vi "Old RoboTaxi VI.vi"() -> ()   [LabVIEW 2022 SP3]
doc: "This example performs writes and reads on a serial port, as directed by the user. You can press the Write and Read buttons, and change the Read Count, while the example is running.\n\nThe parameters set for the serial port must match the parameters of the connected instrument or device. In this example, the Read Count parameter specifies the number of bytes that the serial port reads. If there were more bytes at the port than the specified number, those bytes would not be read. If there were less bytes at the port than the specified number, you would receive a timeout error.\n\nThis example expands upon the flow control options for XON and XOFF, allowing the user to choose those control characters. Also, the user can enable or disable a termination character. Some devices require a termination character in order to identify the end of command strings. Some devices send a termination character to signify the end of data to be read. This example shows how you can end the Read operation once a termination character is detected in the buffer and/or append a termination character at the end of the Write data."
uses:
  Serial - Settings.ctl
  Serial - XON-XOFF Characters.ctl
  Serial - ASCII Characters.ctl
  ESP32-PSOC-State Machine.ctl
  <vilib>/Instr/_visa.llb/VISA Flush IO Buffer Mask.ctl
  <vilib>/Instr/_visa.llb/VISA Configure Serial Port (Instr).vi
panel:
  in  "Stop Driving":bool
  in  "Right":bool
  in  "Left":bool
  in  "Backward":bool
  in  "Forward":bool
  in  "Manual":bool
  in  "Autonomous":bool
  in  "Track 2":bool
  in  "Track 1":bool
  out "error":bool
  out "Connected":bool
  out "Serial Settings:Number of Bytes at Serial Port":u32
  out "Response 2":string
  in  "Toggle LED":bool
  in  "Enum":T1
  in  "Termination Character":u8=10 format="%.0x"
  in  "End Write on Termination Character?":bool=TRUE
  in  "Stop":bool
  out "Read Count":u32=1000
  out "Response":string
  in  "XON/XOFF Characters":T2={"XON"=enum."DC1", "XOFF"=enum."DC3"}
  in  "Serial Settings":T4={"baud rate"=115200, "data bits"=8, "parity"=enum."None", "stop bits"=10, "flow control"=0} {"flow control" items=["None"=0, "XON/XOFF"=1, "RTS/CTS"=2, "DTR/DSR"=4]; "stop bits" items=["1.0"=10, "1.5"=15, "2.0"=20]; "data bits" min=5 max=8 step=1; "baud rate" items=["75"=75, "110"=110, "134"=134, "150"=150, "300"=300, "600"=600, "1200"=1200, "1800"=1800, "2400"=2400, "4800"=4800, "7200"=7200, "9600"=9600, "14400"=14400, "19200"=19200, "28800"=28800, "38400"=38400, "56000"=56000, "57600"=57600, "115200"=115200, "128000"=128000, "230400"=230400]}
  in  "End Read on Termination Character?":bool=TRUE
  in  "VISA resource name":refnum<visa-resource-name>="COM5"
  # "ESP32 Control"
  # "Track Selection"
  # "Driving Mode"
  # "Manual Override"
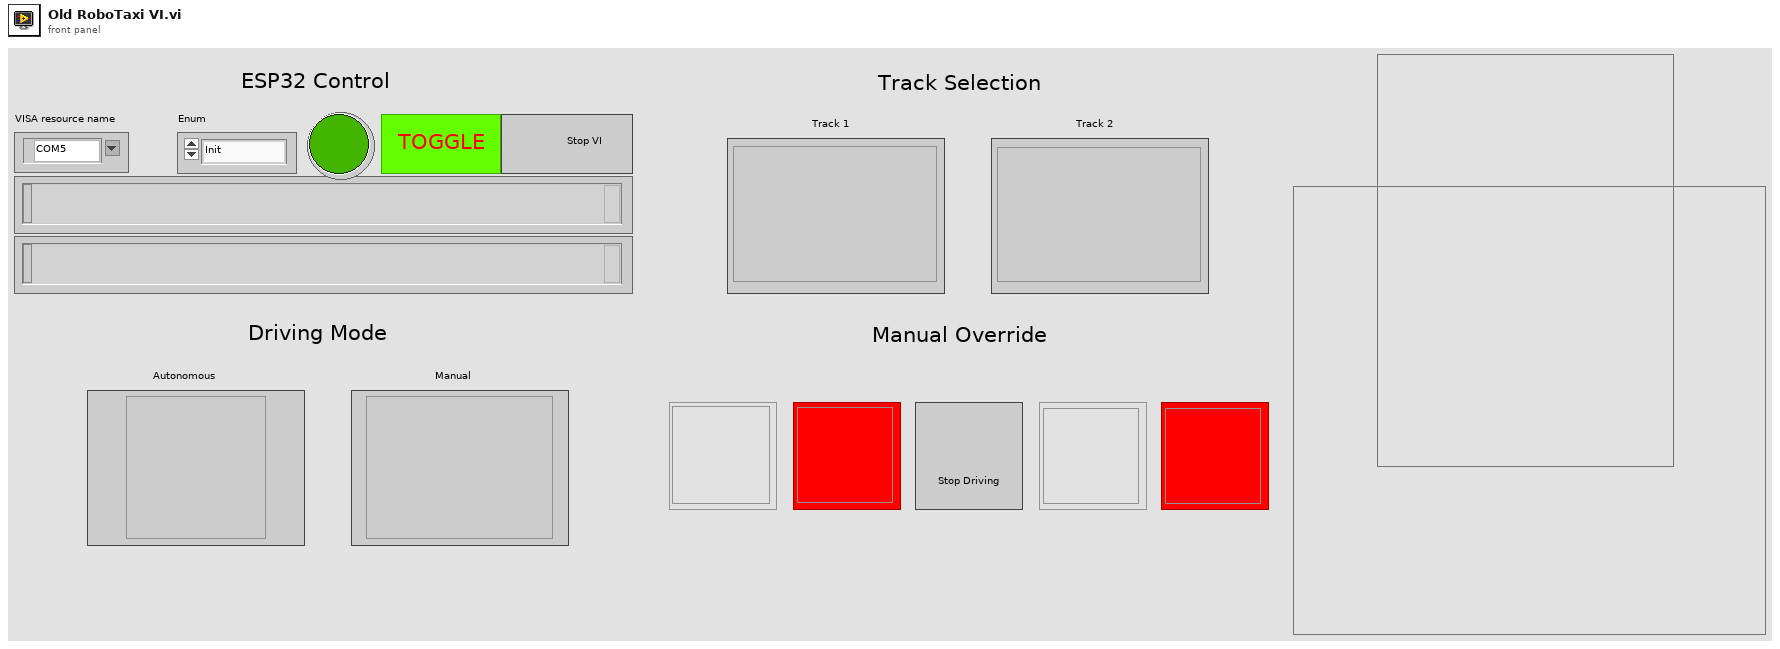
[diagram p1: front panel]
types:
  T1 = typedef "ESP32-PSOC-State Machine.ctl" = enum8{"Init", "Connect", "idle", "send", "wait", "receive", "que", "error", "exit"}
  T2 = typedef "Serial - XON-XOFF Characters.ctl" = cluster{"XON":T3, "XOFF":T3}
  T3 = typedef "Serial - ASCII Characters.ctl" = enum16{"NUL", "SOH", "STX", "ETX", "EOT", "ENQ", "ACK", "BEL", "BS", "HT", "LF", "VT", "FF", "CR", "SO", "SI", "DLE", "DC1", "DC2", "DC3", "DC4", "NAK", "SYN", "ETB", "CAN", "EM", "SUB", "ESC", "FS", "GS", "RS", "US", "SP", "!", "\"", "#", "$", "%", "&", "'", "(", ")", "*", "+", ",", "- (-)", ".", "/", "0", "1", "2", "3", "4", "5", "6", "7", "8", "9", ":", ";", "<", "=", ">", "?", "@", "A", "B", "C", "D", "E", "F", "G", "H", "I", "J", "K", "L", "M", "N", "O", "P", "Q", "R", "S", "T", "U", "V", "W", "X", "Y", "Z", "[", "\\", "]", "^", "_", "`", "a", "b", "c", "d", "e", "f", "g", "h", "i", "j", "k", "l", "m", "n", "o", "p", "q", "r", "s", "t", "u", "v", "w", "x", "y", "z", "{", "|", "}", "~"}
  T4 = typedef "Serial - Settings.ctl" = cluster{"baud rate":u32, "data bits":u16, "parity":enum16{"None", "Odd", "Even", "Mark", "Space"}, "stop bits":u16, "flow control":u16}
  T5 = typedef "VISA Flush IO Buffer Mask.ctl" = u16
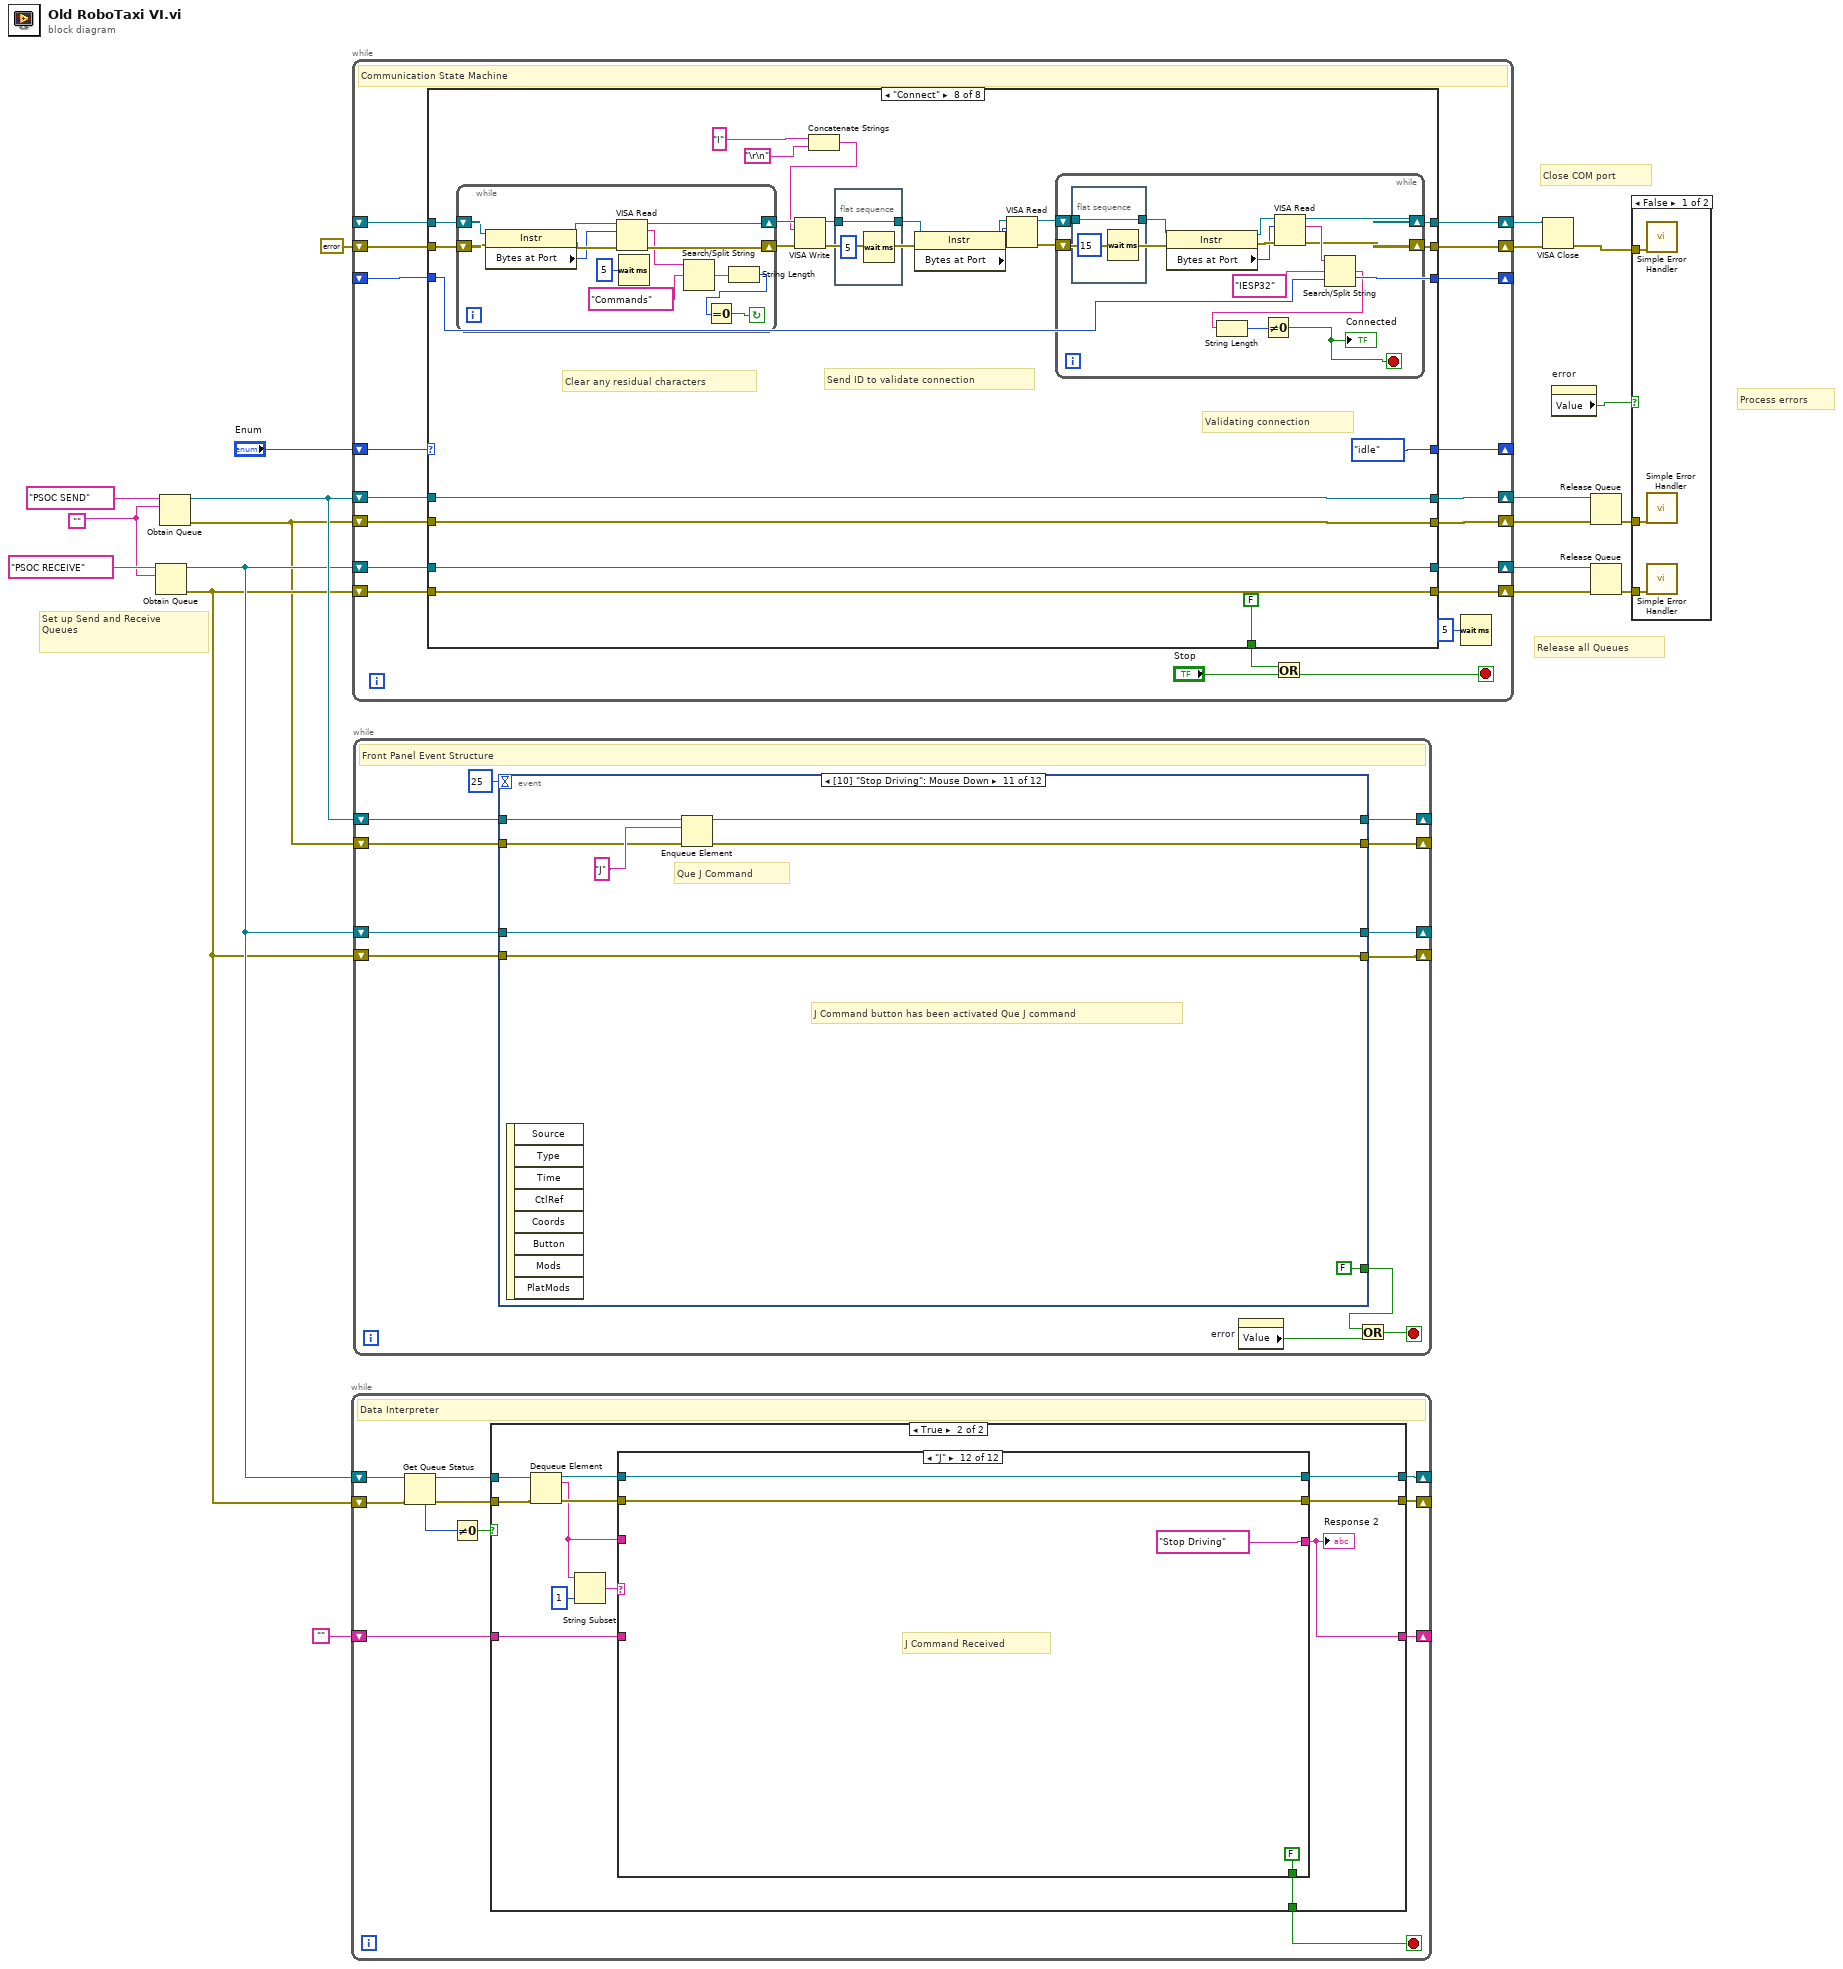
[diagram p0: block diagram]
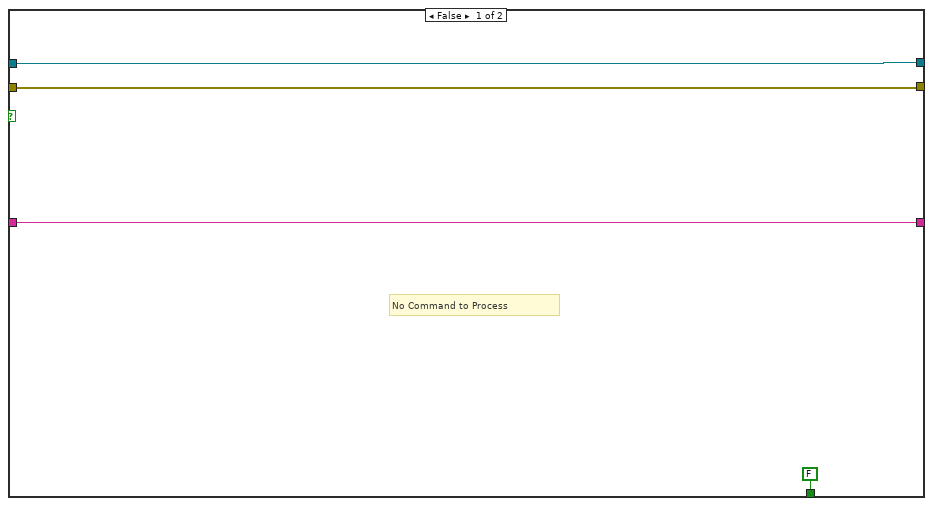
[diagram p3: hidden frame]
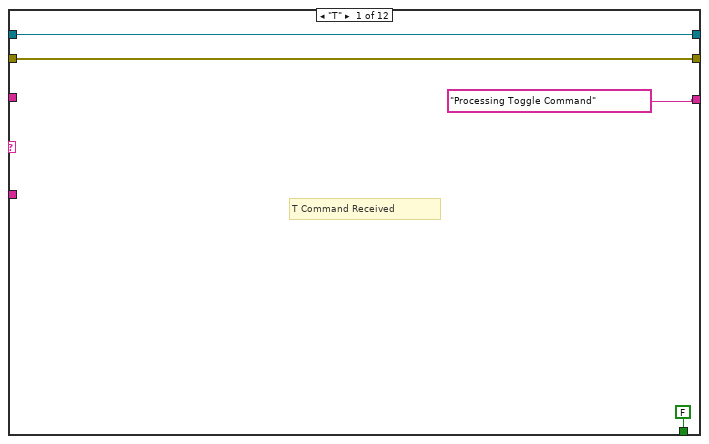
[diagram p4: hidden frame]
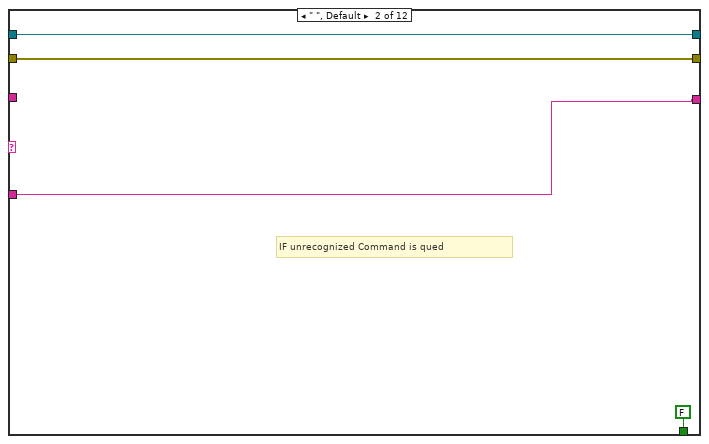
[diagram p5: hidden frame]
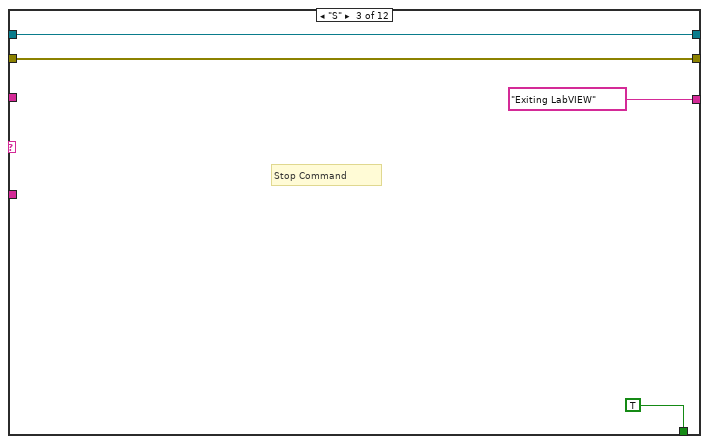
[diagram p6: hidden frame]
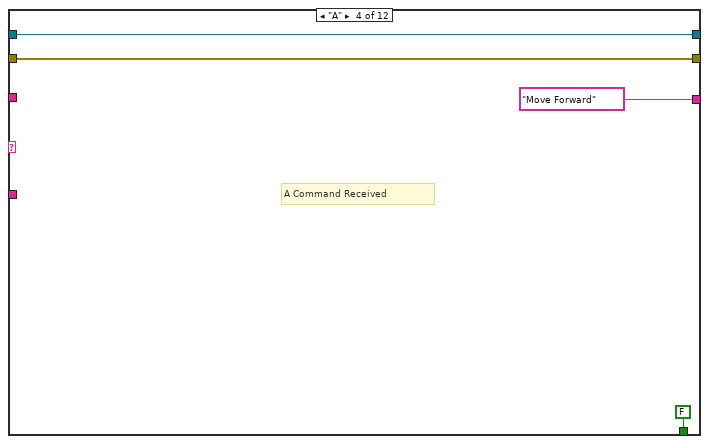
[diagram p7: hidden frame]
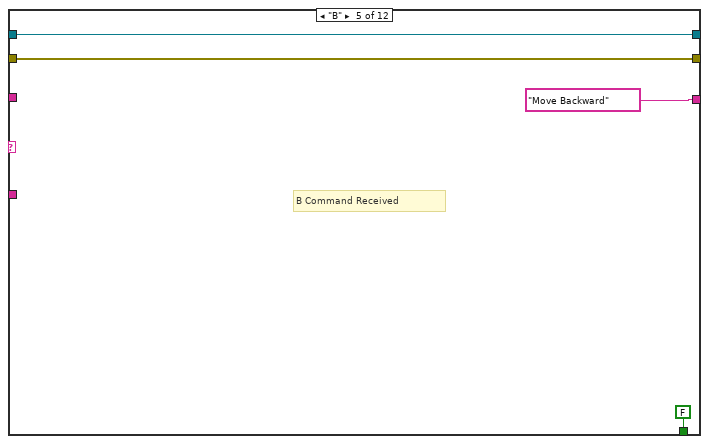
[diagram p8: hidden frame]
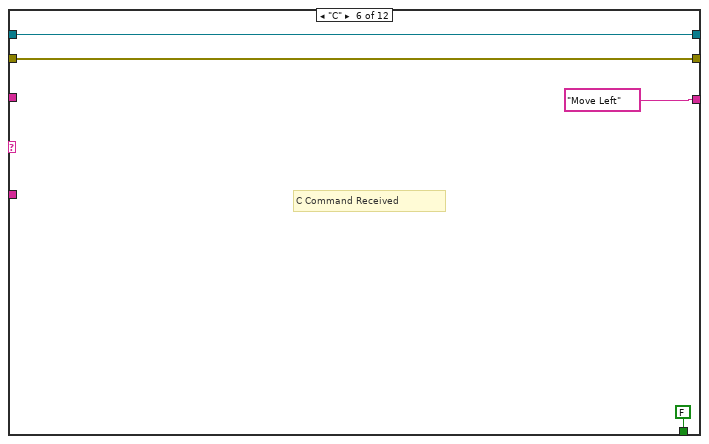
[diagram p9: hidden frame]
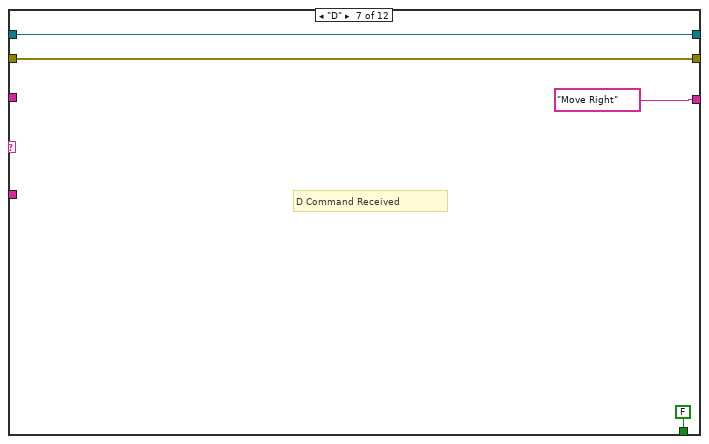
[diagram p10: hidden frame]
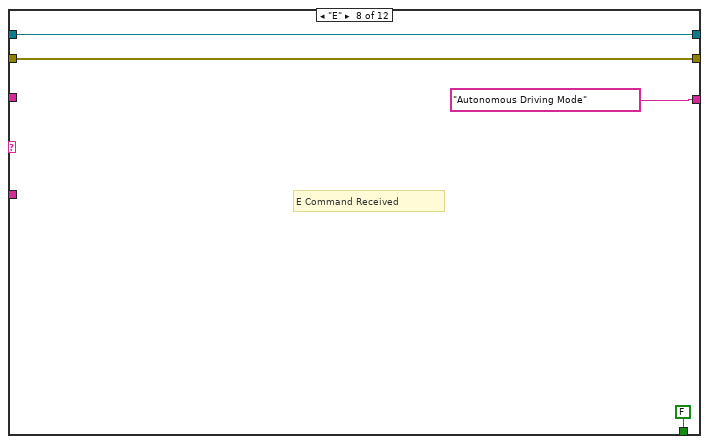
[diagram p11: hidden frame]
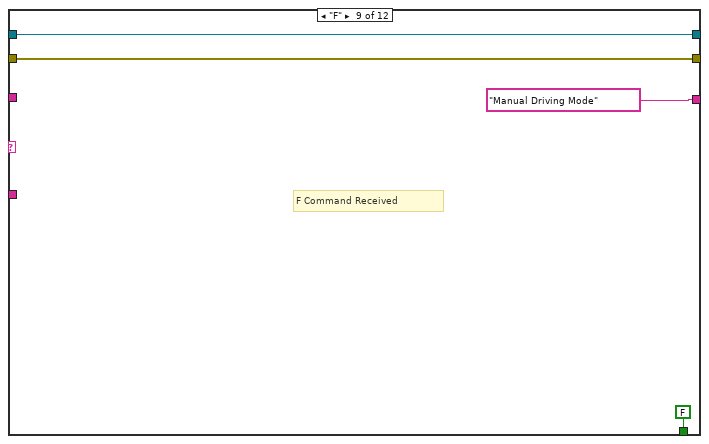
[diagram p12: hidden frame]
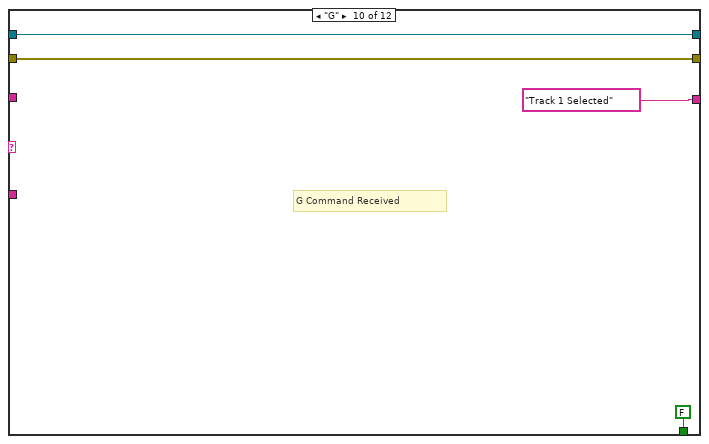
[diagram p13: hidden frame]
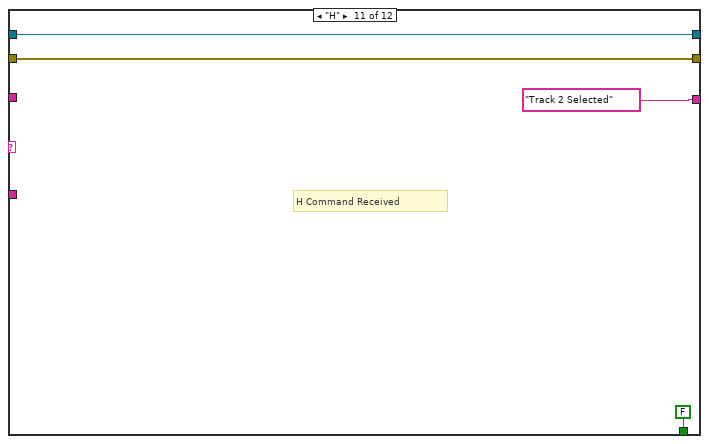
[diagram p14: hidden frame]
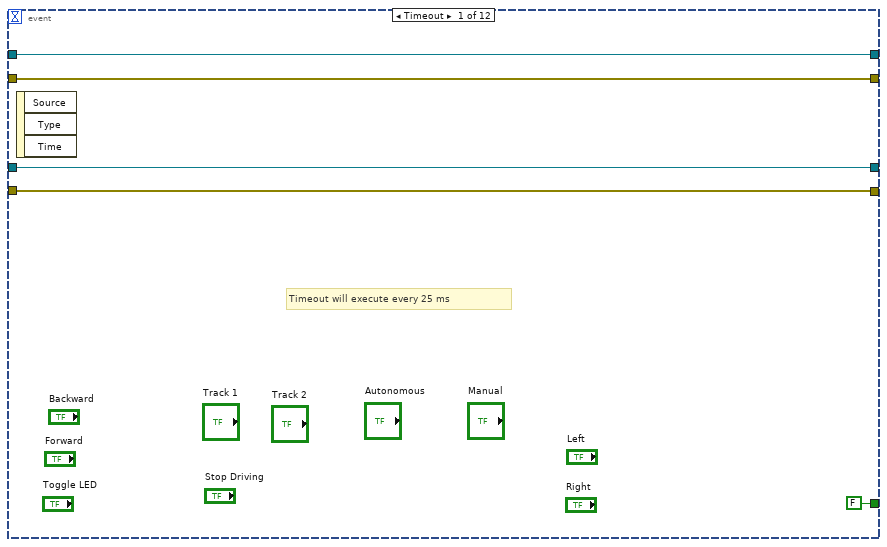
[diagram p15: hidden frame]
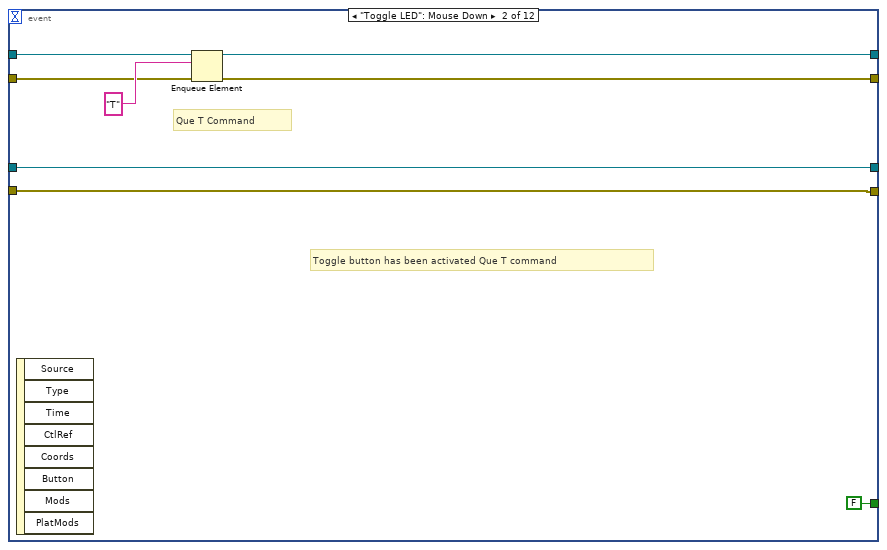
[diagram p16: hidden frame]
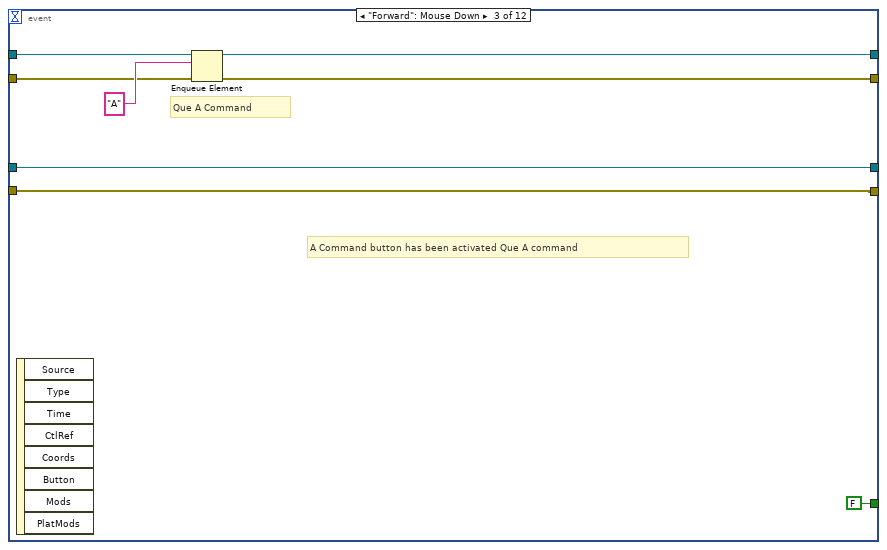
[diagram p17: hidden frame]
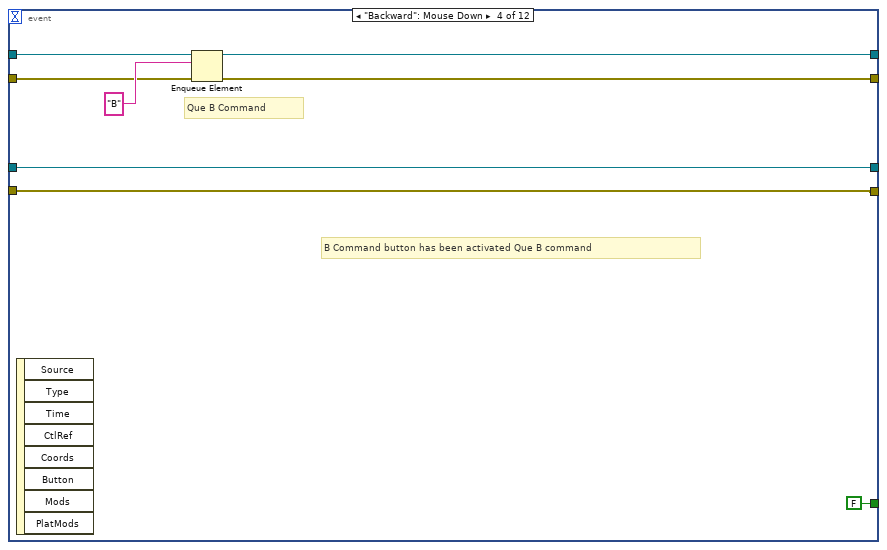
[diagram p18: hidden frame]
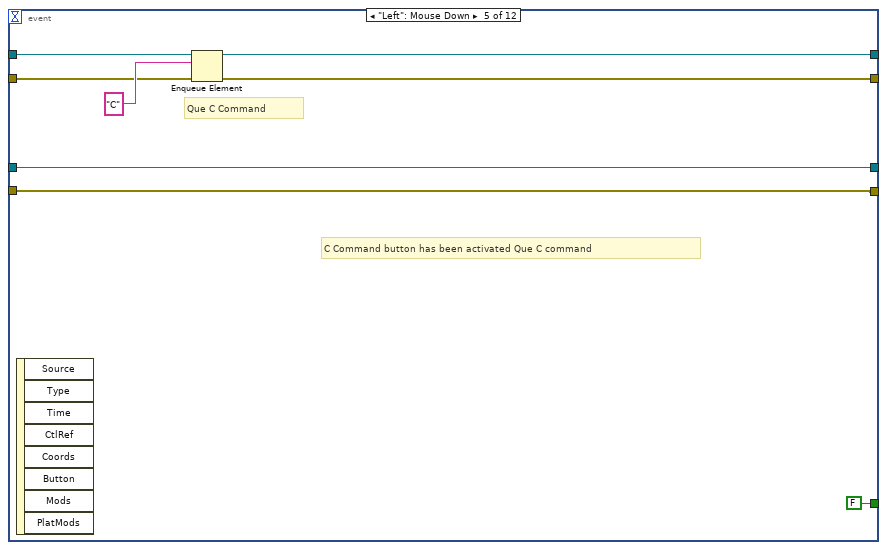
[diagram p19: hidden frame]
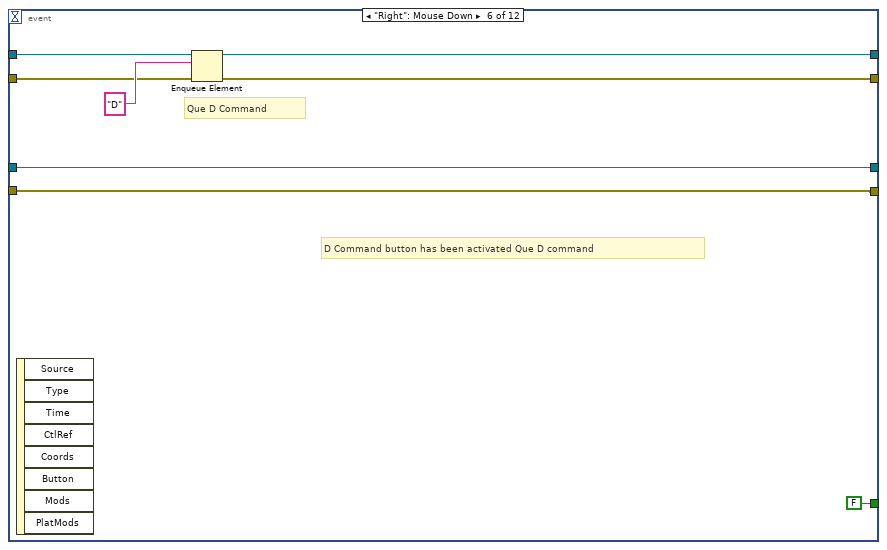
[diagram p20: hidden frame]
diagram:
  w10 = ""
  # "Process errors"
  # "Release all Queues"
  # "Close COM port"
  # "Set up Send and Receive\nQueues"
  n1 = Obtain Queue(name (unnamed)="PSOC RECEIVE", element data type=w10) -> (queue out=w9:refnum<queue>, error out=w8:errorcluster)  [unwired: 3 in, 1 out]
  n2 = Obtain Queue(name (unnamed)="PSOC SEND", element data type=w10) -> (queue out=w12:refnum<queue>, error out=w2:errorcluster)  [unwired: 3 in, 1 out]
  n3 = while {
    shift-right: [w25] -> _
    shift-left: w9 -> [w31]
    shift-right: [w24] -> _
    shift-left: w8 -> [w30]
    shift-right: [w22] -> _
    shift-left: "" -> [w21]
    stop <- w23 stop-if-true
    # "Data Interpreter"
    n4 = Get Queue Status(queue=w31, error in (no error)=w30) -> (queue out=w27:refnum<queue>, error out=w26:errorcluster, # elements in queue=w29:i32)  [unwired: 1 in, 5 out]
    n5 = Not Equal To 0?(x=w29) -> (x != 0?=w28:bool)
    n6 = case shown="True" w28 {
      tunnel: w27 -> [w35 w47]
      tunnel: w26 -> [w34 w46]
      tunnel: [w35 w41] -> w25
      tunnel: [w34 w40] -> w24
      tunnel: [FALSE w39] -> w23
      tunnel: [w32 w37] -> w22
      tunnel: w21 -> [w32 w36]
      frame False {
        # "No Command to Process"
      }
      frame True {
        n7 = Dequeue Element(queue=w47, error in (no error)=w46) -> (queue out=w45:refnum<queue>, element=w38:string, error out=w44:errorcluster)  [unwired: 1 in, 1 out]
        n8 = String Subset(string=w38, length (rest)=1 ("length (rest)")) -> (substring=w42:string)  [unwired: 1 in]
        n9 = case shown="\"J\"" w42 {
          tunnel: w45 -> [w51 w55 w59 w63 w67 w71 w75 w79 w83 w87 w91 w95]
          tunnel: w44 -> [w50 w54 w58 w62 w66 w70 w74 w78 w82 w86 w90 w94]
          tunnel: [w51 w55 w59 w63 w67 w71 w75 w79 w83 w87 w91 w95] -> w41
          tunnel: [w50 w54 w58 w62 w66 w70 w74 w78 w82 w86 w90 w94] -> w40
          tunnel: w38 -> [_ _ _ _ _ _ _ _ _ _ _ _]
          tunnel: [FALSE FALSE TRUE FALSE FALSE FALSE FALSE FALSE FALSE FALSE FALSE FALSE] -> w39
          tunnel: ["Processing Toggle Command" w52 "Exiting LabVIEW" "Move Forward" "Move Backward" "Move Left" "Move Right" "Autonomous Driving Mode" "Manual Driving Mode" "Track 1 Selected" "Track 2 Selected" "Stop Driving"] -> w37
          tunnel: w36 -> [_ w52 _ _ _ _ _ _ _ _ _ _]
          frame "T" {
            # "T Command Received"
          }
          frame " ", Default {
            # "IF unrecognized Command is qued"
          }
          frame "S" {
            # "Stop Command"
          }
          frame "A" {
            # "A Command Received"
          }
          frame "B" {
            # "B Command Received"
          }
          frame "C" {
            # "C Command Received"
          }
          frame "D" {
            # "D Command Received"
          }
          frame "E" {
            # "E Command Received"
          }
          frame "F" {
            # "F Command Received"
          }
          frame "G" {
            # "G Command Received"
          }
          frame "H" {
            # "H Command Received"
          }
          frame "J" {
            # "J Command Received"
          }
        }
        "Response 2" <- w37
      }
    }
  }
  n10 = while {
    shift-right: [w107] -> w20
    shift-left: w12 -> [w115]
    shift-right: [w106] -> w18
    shift-left: w2 -> [w114]
    shift-right: [w105] -> w19
    shift-left: w9 -> [w113]
    shift-right: [w104] -> w15
    shift-left: w8 -> [w112]
    shift-right: [w99] -> _
    shift-left: "Enum" -> [w98]
    shift-right: [w111] -> w14
    shift-left: _ -> [w108]
    shift-right: [w110] -> w13
    shift-left: errorcluster {"status"=FALSE, "code"=0, "source"=""} ("error out") -> [w109]
    shift-right: [w103] -> _
    shift-left: _ -> [w102]
    stop <- w97 stop-if-true
    # "Communication State Machine"
    n11 = case shown="\"Connect\"" w98 {
      selector: w98 -> [_ _ _ _ _ _ w315 _]
      tunnel: [w145 w181 w220 w237 w274 w299 w314 w337] -> w107
      tunnel: [w119 w171 w211 w231 w256 w296 w313 w336] -> w106
      tunnel: [w125 w179 w212 w240 w275 ESP32-PSOC-State_Machine."exit" ("Enum") w315 ESP32-PSOC-State_Machine."idle" ("Enum")] -> w99
      tunnel: w115 -> [w145 w183 w222 w237 w274 w299 w314 w337]
      tunnel: w114 -> [w119 w182 w221 w231 w256 w296 w313 w336]
      tunnel: w113 -> [w146 w177 w219 w234 w269 w298 w312 w335]
      tunnel: w112 -> [w118 w170 w210 w230 w255 w295 w303 w334]
      tunnel: [w127 w174 w206 w239 w264 w301 w318 w339] -> w111
      tunnel: [w121 w172 w207 w232 w257 w297 w317 w340] -> w110
      tunnel: w109 -> [w123 w173 w215 w238 w259 w297 w317 w341]
      tunnel: w108 -> [_ w175 w217 w228 w272 w301 w318 w342]
      tunnel: [w146 w177 w219 w234 w267 w298 w310 w335] -> w105
      tunnel: [w118 w170 w210 w230 w268 w295 w306 w334] -> w104
      tunnel: [u32 0 ("Bytes at Port") w176 w218 w236 w270 w300 w316 w338] -> w103
      tunnel: w102 -> [_ w176 w218 _ w266 w300 w316 w338]
      tunnel: [FALSE FALSE FALSE FALSE FALSE FALSE TRUE FALSE] -> w96
      frame "Init", Default {
        # "Init State ::  Set up Serial COM port"
        # "Set the ASRL End Out property to \"TermChar\" to append a termination character on write."
        n12 = Unbundle By Name("Serial Settings") -> ("baud rate"=w135:u32, "data bits"=w134:u16, "parity"=w133:enum16{"None", "Odd", "Even", "Mark", "Space"}, "stop bits"=w132:u16, "flow control"=w138:u16)
        n13 = Unbundle By Name("XON/XOFF Characters") -> ("XON"=w139:T3, "XOFF"=w140:T3)
        n14 = property on="error" class="Bool (strict)"("Value"=FALSE ("error")) -> ()  [unwired: 2 in, 2 out]
        n15 = property on="Response 2" class="Str"("Value"="") -> ()  [unwired: 2 in, 2 out]
        n16 = call-poly "VISA Configure Serial Port"("VISA resource name"="VISA resource name", "termination char\n(0xA = '\\n' = LF)"="Termination Character", "Enable Termination\nChar (T)"="End Read on Termination Character?", "baud rate (9600)"=w135, "data bits (8)"=w134, "parity (0:none)"=w133, "error in (no error)"=w123, "stop bits (10: 1 bit)"=w132, "flow control (0:none)"=w138) -> ("VISA resource name out"=w131:refnum<visa-resource-name>, "error out"=w130:errorcluster)  [unwired: 1 in, 4 out]
        n17 = case shown="Default" w138 {
          tunnel: [w158 w167] -> w141
          tunnel: [w159 w166] -> w142
          tunnel: w130 -> [w158 w165]
          tunnel: w131 -> [w159 w164]
          tunnel: w139 -> [_ w163]
          tunnel: w140 -> [_ w162]
          frame Default {
          }
          frame 1 {
            n18 = To Unsigned Byte Integer(number=w162) -> (unsigned 8bit integer=w161:u8)
            n19 = To Unsigned Byte Integer(number=w163) -> (unsigned 8bit integer=w160:u8)
            n20 = property class="Instr"(reference=w164, error in=w165, "Serial Settings:Flow Control XON Character"=w160, "Serial Settings:Flow Control XOFF Character"=w161) -> (reference out=w166:refnum<visa-resource-name>, error out=w167:errorcluster)
          }
        }
        n21 = case shown="True" "End Write on Termination Character?" {
          tunnel: w142 -> [w149 w157]
          tunnel: w141 -> [w150 w156]
          tunnel: [w149 w155] -> w127
          tunnel: [w150 w154] -> w121
          tunnel: "Termination Character" -> [_ w152]
          frame False {
          }
          frame True {
            w153 = u16 2 items=["None", "LastBit", "TermChar", "Break"] ("Serial Settings:Serial End Mode for Writes")
            n22 = property class="Instr"(reference=w157, error in=w156, "Serial Settings:End Mode for Writes"=w153, "Message Based Settings:Send End Enable"=TRUE, "Message Based Settings:Termination Character"=w152) -> (reference out=w155:refnum<visa-resource-name>, error out=w154:errorcluster)
          }
        }
        n23 = Or(x=w118, y=w119) -> (x .or. y?=w120:bool)
        n24 = Or(x=w121, y=w120) -> (x .or. y?=w122:bool)
        n25 = case shown="False" w122 {
          tunnel: [ESP32-PSOC-State_Machine."Connect" ("Enum") ESP32-PSOC-State_Machine."error" ("Enum")] -> w125
          frame False {
          }
          frame True {
          }
        }
      }
      frame "idle" {
        # "Wait until Command is in queue"
        n26 = Get Queue Status(queue=w183, error in (no error)=w182) -> (queue out=w181:refnum<queue>, error out=w171:errorcluster, # elements in queue=w180:i32)  [unwired: 1 in, 5 out]
        n27 = Not Equal To 0?(x=w180) -> (x != 0?=w178:bool)
        n28 = while {
          tunnel: w175 -> [w196]
          tunnel: [w192] -> w174
          tunnel: w173 -> [w195]
          tunnel: [w190] -> w172
          stop <- w194 continue-if-true
          # "Clear Boot Message"
          n29 = property class="Instr"(reference=w196, error in=w195) -> (reference out=w193:refnum<visa-resource-name>, error out=w191:errorcluster, "Serial Settings:Number of Bytes at Serial Port"=w189:u32)
          "Serial Settings:Number of Bytes at Serial Port" <- w189
          n30 = Not Equal To 0?(x=w189) -> (x != 0?=w194:bool)
          n31 = VISA Read(VISA resource name=w193, byte count=w189, error in (no error)=w191) -> (VISA resource name out=w192:refnum<visa-resource-name>, error out=w190:errorcluster)  [unwired: 2 out]
        }
        n32 = Compound Arithmetic op=OR(w172, w171, w170) -> (w169:bool)
        n33 = case shown="True" w169 {
          tunnel: [w185 ESP32-PSOC-State_Machine."error" ("Enum")] -> w179
          tunnel: w178 -> [w184 _]
          frame False {
            n34 = case shown="False" w184 {
              tunnel: [ESP32-PSOC-State_Machine."idle" ("Enum") ESP32-PSOC-State_Machine."send" ("Enum")] -> w185
              frame False {
              }
              frame True {
              }
            }
          }
          frame True {
          }
        }
      }
      frame "send" {
        w213 = T5 64 items=["Flush Receive Buffer"=16, "Write Transmit Buffer to Device"=32, "Flush Receive Buffer (No I/O)"=64, "Flush Transmit Buffer"=128] ("Mask")
        # "Read and Discard Echo Command"
        # "Wait for Response"
        # "Send Command"
        n35 = Dequeue Element(queue=w222, error in (no error)=w221) -> (queue out=w220:refnum<queue>, element=w200:string, error out=w211:errorcluster)  [unwired: 1 in, 1 out]
        n36 = VISA Flush I/O Buffer(VISA resource name=w217, mask (16)=w213, error in (no error)=w215) -> (VISA resource name out=w216:refnum<visa-resource-name>, error out=w214:errorcluster)
        n37 = Concatenate Strings(w200, "\r\n") -> (w199:string)
        n38 = VISA Write(VISA resource name=w216, write buffer=w199, error in (no error)=w214) -> (VISA resource name out=w198:refnum<visa-resource-name>, error out=w204:errorcluster)  [unwired: 1 out]
        n39 = flat-sequence {
          tunnel: w198 -> [w224]
          tunnel: [w224] -> w197
          frame #0 {
            n40 = Wait (ms)(milliseconds to wait=u32 15) -> ()  [unwired: 1 out]
          }
        }
        n41 = property class="Instr"(reference=w197, error in=w204) -> (reference out=w205:refnum<visa-resource-name>, error out=w203:errorcluster, "Serial Settings:Number of Bytes at Serial Port"=w202:u32)
        n42 = VISA Read(VISA resource name=w205, byte count=w202, error in (no error)=w203) -> (VISA resource name out=w206:refnum<visa-resource-name>, error out=w207:errorcluster)  [unwired: 2 out]
        n43 = Compound Arithmetic op=OR(w207, w211, w210) -> (w209:bool)
        n44 = case shown="False" w209 {
          tunnel: [ESP32-PSOC-State_Machine."wait" ("Enum") ESP32-PSOC-State_Machine."error" ("Enum")] -> w212
          frame False {
          }
          frame True {
          }
        }
      }
      frame "wait" {
        # "Wait for actual Response"
        n45 = flat-sequence {
          tunnel: w228 -> [w242]
          tunnel: [w242] -> w227
          frame #0 {
            n46 = Wait (ms)(milliseconds to wait=u32 15) -> ()  [unwired: 1 out]
          }
        }
        n47 = property class="Instr"(reference=w227, error in=w238) -> (reference out=w239:refnum<visa-resource-name>, error out=w232:errorcluster, "Serial Settings:Number of Bytes at Serial Port"=w236:u32)
        n48 = Not Equal To 0?(x=w236) -> (x != 0?=w235:bool)
        n49 = Compound Arithmetic op=OR(w232, w231, w230) -> (w233:bool)
        n50 = case shown="False" w233 {
          tunnel: [w244 ESP32-PSOC-State_Machine."error" ("Enum")] -> w240
          tunnel: w235 -> [w243 _]
          frame False {
            n51 = case shown="True" w243 {
              tunnel: [ESP32-PSOC-State_Machine."wait" ("Enum") ESP32-PSOC-State_Machine."receive" ("Enum")] -> w244
              frame False {
              }
              frame True {
              }
            }
          }
          frame True {
          }
        }
      }
      frame "receive" {
        # "Process Response and Display"
        # "Read Response"
        n52 = VISA Read(VISA resource name=w272, byte count=w266, error in (no error)=w259) -> (VISA resource name out=w265:refnum<visa-resource-name>, read buffer=w261:string, error out=w271:errorcluster)  [unwired: 1 out]
        n53 = String To Byte Array(string=w261) -> (unsigned byte array=w260:u8[])
        n54 = property class="Instr"(reference=w265, error in=w271) -> (reference out=w264:refnum<visa-resource-name>, error out=w258:errorcluster, "Serial Settings:Number of Bytes at Serial Port"=w270:u32)
        n55 = Index Array(array=w260, index=0) -> (element=w252:u8)
        n56 = Equal?(x=w252, y=u8 13) -> (x = y?=w250:bool)
        n57 = Equal?(x=w252, y=u8 10) -> (x = y?=w249:bool)
        n58 = Not Or(1:w249, 2:w250) -> (0:w248:bool)
        n59 = Not Equal To 0?(x=w270) -> (x != 0?=w273:bool)
        n60 = case shown="True" w248 {
          tunnel: w260 -> [_ w290]
          tunnel: w258 -> [w281 w283]
          tunnel: [w281 w282] -> w257
          frame False {
          }
          frame True {
            n61 = Delete From Array(array=w290, length=1, index=0) -> (array with subset deleted=w287:u8[])  [unwired: 1 out]
            n62 = property on="Response" class="Str"(error in=w283, "Value"="") -> (error out=w285:errorcluster)  [unwired: 1 in, 1 out]
            n63 = Byte Array To String(unsigned byte array=w287) -> (string=w284:string)
            n64 = property on="Response" class="Str"(error in=w285, "Value"=w284) -> (error out=w282:errorcluster)  [unwired: 1 in, 1 out]
          }
        }
        n65 = Compound Arithmetic op=OR(w257, w256, w255) -> (w254:bool)
        n66 = Enqueue Element(queue=w269, element=w261, error in (no error)=w255) -> (queue out=w267:refnum<queue>, error out=w268:errorcluster)  [unwired: 1 in, 1 out]
        n67 = case shown="False" w254 {
          tunnel: [w277 ESP32-PSOC-State_Machine."error" ("Enum")] -> w275
          tunnel: w273 -> [w276 _]
          frame False {
            n68 = case shown="False" w276 {
              tunnel: [ESP32-PSOC-State_Machine."idle" ("Enum") ESP32-PSOC-State_Machine."receive" ("Enum")] -> w277
              frame False {
              }
              frame True {
              }
            }
          }
          frame True {
          }
        }
        "Read Count" <- w266
      }
      frame "error" {
        # "Process any error"
        n69 = Build Array(w297, w296, w295) -> (w294:errorcluster[])
        n70 = for {
          tunnel: w294 -> [w302] mode=indexing
          n71 = call <vilib>:"General Error Handler.vi"("error in (no error)"=w302) -> ()  [unwired: 10 in, 5 out]
        }
        "error" <- TRUE ("error")
      }
      frame "exit" {
        # "Exit due to error"
        n72 = Enqueue Element(queue=w312, element="S", error in (no error)=w303) -> (queue out=w310:refnum<queue>, error out=w308:errorcluster)  [unwired: 1 in, 1 out]
        n73 = property on="Connected" class="Bool (strict)"(error in=w308, "Value"=FALSE ("Connected")) -> (error out=w307:errorcluster)  [unwired: 1 in, 1 out]
        n74 = property on="Response" class="Str"(error in=w307, "Value"="") -> (error out=w306:errorcluster)  [unwired: 1 in, 1 out]
      }
      frame "Connect" {
        # "Validating connection"
        # "Send ID to validate connection"
        # "Clear any residual characters"
        n75 = while {
          shift-right: [w366] -> w330
          shift-left: w341 -> [w372]
          shift-right: [w365] -> w331
          shift-left: w342 -> [w371]
          stop <- w370 continue-if-true
          n76 = property class="Instr"(reference=w371, error in=w372) -> (reference out=w368:refnum<visa-resource-name>, error out=w367:errorcluster, "Bytes at Port"=w364:u32)
          n77 = VISA Read(VISA resource name=w368, byte count=w364, error in (no error)=w367) -> (VISA resource name out=w365:refnum<visa-resource-name>, read buffer=w363:string, error out=w366:errorcluster)  [unwired: 1 out]
          n78 = Wait (ms)(milliseconds to wait=u32 5) -> ()  [unwired: 1 out]
          n79 = Search/Split String(string=w363, search string/char (-)="Commands") -> (match + rest of string=w361:string)  [unwired: 1 in, 2 out]
          n80 = String Length(string=w361) -> (length=w360:i32)
          n81 = Equal To 0?(x=w360) -> (x = 0?=w370:bool)
        }
        n82 = Concatenate Strings("I" ("write buffer"), "\r\n") -> (w319:string)
        n83 = VISA Write(VISA resource name=w331, write buffer=w319, error in (no error)=w330) -> (VISA resource name out=w325:refnum<visa-resource-name>, error out=w329:errorcluster)  [unwired: 1 out]
        n84 = flat-sequence {
          tunnel: w325 -> [w359]
          tunnel: [w359] -> w324
          frame #0 {
            n85 = Wait (ms)(milliseconds to wait=u32 5) -> ()  [unwired: 1 out]
          }
        }
        n86 = property class="Instr"(reference=w324, error in=w329) -> (reference out=w327:refnum<visa-resource-name>, error out=w328:errorcluster, "Bytes at Port"=w326:u32)
        n87 = VISA Read(VISA resource name=w327, byte count=w326, error in (no error)=w328) -> (VISA resource name out=w322:refnum<visa-resource-name>, error out=w323:errorcluster)  [unwired: 2 out]
        n88 = while {
          shift-right: [w346] -> w340
          shift-left: w323 -> [w352]
          shift-right: [w347] -> w339
          shift-left: w322 -> [w345]
          stop <- w343 stop-if-true
          n89 = flat-sequence {
            tunnel: w345 -> [w357]
            tunnel: [w357] -> w344
            frame #0 {
              n90 = Wait (ms)(milliseconds to wait=u32 15) -> ()  [unwired: 1 out]
            }
          }
          n91 = property class="Instr"(reference=w344, error in=w352) -> (reference out=w350:refnum<visa-resource-name>, error out=w351:errorcluster, "Bytes at Port"=w349:u32)
          n92 = VISA Read(VISA resource name=w350, byte count=w349, error in (no error)=w351) -> (VISA resource name out=w347:refnum<visa-resource-name>, read buffer=w348:string, error out=w346:errorcluster)  [unwired: 1 out]
          n93 = Search/Split String(string=w348, search string/char (-)="IESP32") -> (match + rest of string=w354:string)  [unwired: 1 in, 2 out]
          n94 = String Length(string=w354) -> (length=w353:i32)
          n95 = Not Equal To 0?(x=w353) -> (x != 0?=w343:bool)
          "Connected" <- w343
        }
      }
    }
    n96 = Or(x=w96, y="Stop") -> (x .or. y?=w97:bool)
    n97 = Wait (ms)(milliseconds to wait=u32 5) -> ()  [unwired: 1 out]
  }
  n98 = while {
    shift-right: [w381] -> _
    shift-left: w12 -> [w382]
    shift-right: [w380] -> _
    shift-left: w2 -> [w383]
    shift-right: [w376] -> _
    shift-left: w9 -> [w379]
    shift-right: [w377] -> _
    shift-left: w8 -> [w378]
    stop <- w373 stop-if-true
    # "Front Panel Event Structure"
    n99 = event shown="[10] \"Stop Driving\": Mouse Down" {
      selector: _ -> [_ _ _ _ _ _ _ _ _ _ _ _]
      dyn-events: _ -> [_ _ _ _ _ _ _ _ _ _ _ _]
      timeout: 25 -> [_ _ _ _ _ _ _ _ _ _ _ _]
      tunnel: w383 -> [w387 w395 w403 w411 w419 w427 w435 w443 w451 w459 w467 w479]
      tunnel: w382 -> [w388 w397 w405 w413 w421 w429 w437 w445 w453 w461 w469 w480]
      tunnel: [w388 w394 w402 w410 w418 w426 w434 w442 w450 w458 w466 w480] -> w381
      tunnel: [w387 w393 w401 w409 w417 w425 w433 w441 w449 w457 w465 w479] -> w380
      tunnel: [FALSE FALSE FALSE FALSE FALSE FALSE FALSE FALSE FALSE FALSE FALSE TRUE] -> w375
      tunnel: w379 -> [w386 w391 w399 w407 w415 w423 w431 w439 w447 w455 w463 w478]
      tunnel: w378 -> [w385 w390 w398 w406 w414 w422 w430 w438 w446 w454 w462 w476]
      tunnel: [w385 w390 w398 w406 w414 w422 w430 w438 w446 w454 w462 w471] -> w377
      tunnel: [w386 w391 w399 w407 w415 w423 w431 w439 w447 w455 w463 w475] -> w376
      event Timeout {
        # "Timeout will execute every 25 ms"
        n100 = event-data() -> ()  [unwired: 1 in, 3 out]
      }
      event "Toggle LED": Mouse Down {
        # "Que T Command"
        # "Toggle button has been activated Que T command"
        n101 = event-data() -> ()  [unwired: 1 in, 8 out]
        n102 = Enqueue Element(queue=w397, element="T", error in (no error)=w395) -> (queue out=w394:refnum<queue>, error out=w393:errorcluster)  [unwired: 1 in, 1 out]
      }
      event "Forward": Mouse Down {
        # "Que A Command"
        # "A Command button has been activated Que A command"
        n103 = event-data() -> ()  [unwired: 1 in, 8 out]
        n104 = Enqueue Element(queue=w405, element="A", error in (no error)=w403) -> (queue out=w402:refnum<queue>, error out=w401:errorcluster)  [unwired: 1 in, 1 out]
      }
      event "Backward": Mouse Down {
        # "Que B Command"
        # "B Command button has been activated Que B command"
        n105 = event-data() -> ()  [unwired: 1 in, 8 out]
        n106 = Enqueue Element(queue=w413, element="B", error in (no error)=w411) -> (queue out=w410:refnum<queue>, error out=w409:errorcluster)  [unwired: 1 in, 1 out]
      }
      event "Left": Mouse Down {
        # "Que C Command"
        # "C Command button has been activated Que C command"
        n107 = event-data() -> ()  [unwired: 1 in, 8 out]
        n108 = Enqueue Element(queue=w421, element="C", error in (no error)=w419) -> (queue out=w418:refnum<queue>, error out=w417:errorcluster)  [unwired: 1 in, 1 out]
      }
      event "Right": Mouse Down {
        # "Que D Command"
        # "D Command button has been activated Que D command"
        n109 = event-data() -> ()  [unwired: 1 in, 8 out]
        n110 = Enqueue Element(queue=w429, element="D", error in (no error)=w427) -> (queue out=w426:refnum<queue>, error out=w425:errorcluster)  [unwired: 1 in, 1 out]
      }
      event "Autonomous": Mouse Down {
        # "Que E Command"
        # "E Command button has been activated Que E command"
        n111 = event-data() -> ()  [unwired: 1 in, 8 out]
        n112 = Enqueue Element(queue=w437, element="E", error in (no error)=w435) -> (queue out=w434:refnum<queue>, error out=w433:errorcluster)  [unwired: 1 in, 1 out]
      }
      event "Manual": Mouse Down {
        # "Que F Command"
        # "F Command button has been activated Que F command"
        n113 = event-data() -> ()  [unwired: 1 in, 8 out]
        n114 = Enqueue Element(queue=w445, element="F", error in (no error)=w443) -> (queue out=w442:refnum<queue>, error out=w441:errorcluster)  [unwired: 1 in, 1 out]
      }
      event "Track 1": Mouse Down {
        # "Que G Command"
        # "G Command button has been activated Que G command"
        n115 = event-data() -> ()  [unwired: 1 in, 8 out]
        n116 = Enqueue Element(queue=w453, element="G", error in (no error)=w451) -> (queue out=w450:refnum<queue>, error out=w449:errorcluster)  [unwired: 1 in, 1 out]
      }
      event "Track 2": Mouse Down {
        # "Que H Command"
        # "H Command button has been activated Que H command"
        n117 = event-data() -> ()  [unwired: 1 in, 8 out]
        n118 = Enqueue Element(queue=w461, element="H", error in (no error)=w459) -> (queue out=w458:refnum<queue>, error out=w457:errorcluster)  [unwired: 1 in, 1 out]
      }
      event "Stop Driving": Mouse Down {
        # "Que J Command"
        # "J Command button has been activated Que J command"
        n119 = event-data() -> ()  [unwired: 1 in, 8 out]
        n120 = Enqueue Element(queue=w469, element="J", error in (no error)=w467) -> (queue out=w466:refnum<queue>, error out=w465:errorcluster)  [unwired: 1 in, 1 out]
      }
      event "Stop": Value Change {
        # "Stop Application"
        n121 = event-data() -> ()  [unwired: 1 in, 6 out]
        n122 = Enqueue Element(queue=w478, element="S", error in (no error)=w476) -> (queue out=w475:refnum<queue>, error out=w474:errorcluster)  [unwired: 1 in, 1 out]
        n123 = property on="Connected" class="Bool (strict)"(error in=w474, "Value"=FALSE ("Connected")) -> (error out=w472:errorcluster)  [unwired: 1 in, 1 out]
        n124 = property on="Response" class="Str"(error in=w472, "Value"="") -> (error out=w471:errorcluster)  [unwired: 1 in, 1 out]
      }
    }
    n125 = property on="error" class="Bool (strict)"() -> ("Value"=w374:bool)  [unwired: 2 in, 2 out]
    n126 = Or(x=w375, y=w374) -> (x .or. y?=w373:bool)
  }
  n127 = VISA Close(VISA resource name=w14, error in (no error)=w13) -> (error out=w5:errorcluster)
  n128 = property on="error" class="Bool (strict)"() -> ("Value"=w1:bool)  [unwired: 2 in, 2 out]
  n129 = Release Queue(queue=w20, error in (no error)=w18) -> (error out=w4:errorcluster)  [unwired: 1 in, 2 out]
  n130 = Release Queue(queue=w19, error in (no error)=w15) -> (error out=w3:errorcluster)  [unwired: 1 in, 2 out]
  n131 = case shown="False" w1 {
    tunnel: w5 -> [w484 _]
    tunnel: w4 -> [w483 _]
    tunnel: w3 -> [w482 _]
    frame False {
      n132 = call <vilib>:"Simple Error Handler.vi"("error in (no error)"=w484) -> ()  [unwired: 1 in, 8 out]
      n133 = call <vilib>:"Simple Error Handler.vi"("error in (no error)"=w483) -> ()  [unwired: 1 in, 8 out]
      n134 = call <vilib>:"Simple Error Handler.vi"("error in (no error)"=w482) -> ()  [unwired: 1 in, 8 out]
    }
    frame True {
    }
  }
